vi "Build S1F1 Message Example.vi"(8 "error in":errorcluster) -> (0 "error out":errorcluster, 3 "SECS Packet":T1)   [LabVIEW 2016]
uses:
  Com/SECS Equipment/Data Def/Com_SECS Equipment _SECS Packet.ctl
  Com/SECS Equipment/Data Def/Com_SECS Equipment _Message Type.ctl
  Com/SECS Equipment/Data Def/Com_SECS Equipment _Protocol Type.ctl
  Com/SECS Equipment/Data Def/Com_SECS Equipment _Stream Type.ctl
  Com/SECS Equipment/Data Def/Com_SECS Equipment _Build Message Setting.ctl
  Com/SECS Equipment/Data Message/Com_SECS Equipment _Data Message_List.vi
  Com/SECS Equipment/Data Message/Com_SECS Equipment _Data Message_Boolean.vi
  Com/SECS Equipment/Data Message/Com_SECS Equipment _Data Message_F4.vi
  Com/SECS Equipment/Data Message/Com_SECS Equipment _Data Message_F8.vi
  Com/SECS Equipment/Data Message/Com_SECS Equipment _Data Message_Binary.vi
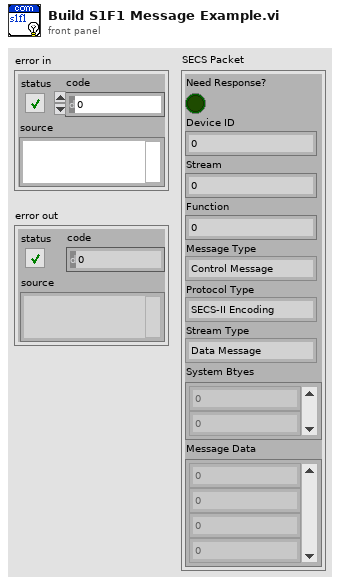
[diagram p1: front panel]
types:
  T1 = typedef "Com_SECS Equipment _SECS Packet.ctl" = cluster{"Need Response?":bool, "Device ID":u16, "Stream":u8, "Function":u8, "Message Type":T2, "Protocol Type":T3, "Stream Type":T4, "System Btyes":u8[], "Message Data":u8[]}
  T2 = typedef "Com_SECS Equipment _Message Type.ctl" = enum16{"Control Message", "Data Message"}
  T3 = typedef "Com_SECS Equipment _Protocol Type.ctl" = enum16{"SECS-II Encoding", "Reserved"}
  T4 = typedef "Com_SECS Equipment _Stream Type.ctl" = enum16{"Data Message", "Select.req", "Select.rsp", "Deselect.req", "Deselect.rsp", "Linktest.req", "Linktest.rsp", "Reject.req", "Separate.req", "Reserve"}
  T5 = typedef "Com_SECS Equipment _Build Message Setting.ctl" = cluster{"Stream":u8, "Function":u8, "Need Response?":bool}
  T6 = typedef "Com_SECS Equipment _Message Data.ctl" = cluster{"Index":i32, "Data Item Format":T7, "Format Code":T8, "Parent Index":i32, "Child Index":i32[], "Data":variant}
  T7 = typedef "Com_SECS Equipment _Data Item Format.ctl" = enum16{"Data Type", "Value"}
  T8 = typedef "Com_SECS Equipment _Format Code.ctl" = enum16{"L", "A", "B", "Boolean", "J", "I1", "I2", "I4", "I8", "U1", "U2", "U4", "U8", "F4", "F8", "Char"}
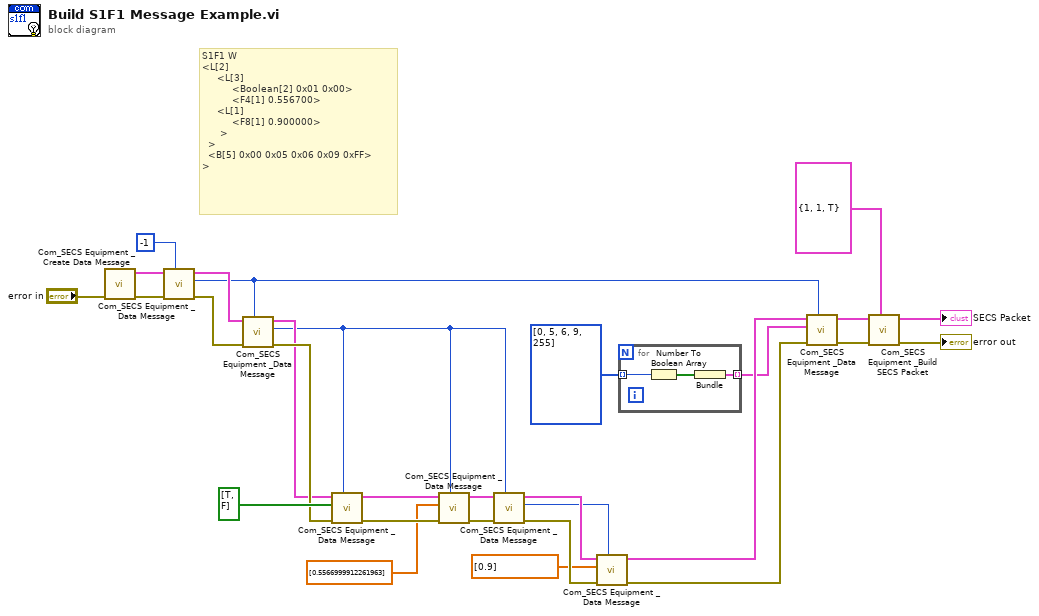
[diagram p0: block diagram]
diagram:
  # "S1F1 W\n<L[2]\n     <L[3]\n          <Boolean[2] 0x01 0x00>\n          <F4[1] 0.556700>\n     <L[1]\n          <F8[1] 0.900000>\n      >\n  >\n  <B[5] 0x00 0x05 0x06 0x09 0xFF>\n>"
  n1 = call "Com_SECS Equipment _Create Data Message.vi"("error in"="error in") -> ("error out"=w29:errorcluster, "Message Data"=w28:T6[])  [unwired: 9 in]
  n2 = call-poly "Com_SECS Equipment _Data Message.vi"("Parent Index"=-1, "error in"=w29, "Message Data In"=w28) -> ("error out"=w23:errorcluster, "Index"=w3:i32, "Message Data Out"=w22:T6[])  [unwired: 6 in]
  n3 = call-poly "Com_SECS Equipment _Data Message.vi"("Parent Index"=w3, "error in"=w23, "Message Data In"=w22) -> ("error out"=w21:errorcluster, "Index"=w2:i32, "Message Data Out"=w20:T6[])  [unwired: 6 in]
  n4 = call-poly "Com_SECS Equipment _Data Message.vi"("Parent Index"=w2, "error in"=w21, "Data"=bool[] [TRUE, FALSE], "Message Data In"=w20) -> ("error out"=w24:errorcluster, "Message Data Out"=w25:T6[])  [unwired: 6 in]
  n5 = call-poly "Com_SECS Equipment _Data Message.vi"("Parent Index"=w2, "error in"=w24, "Data"=sgl[] [0.5567], "Message Data In"=w25) -> ("error out"=w19:errorcluster, "Message Data Out"=w18:T6[])  [unwired: 6 in]
  n6 = call-poly "Com_SECS Equipment _Data Message.vi"("Parent Index"=w2, "error in"=w19, "Message Data In"=w18) -> ("error out"=w16:errorcluster, "Index"=w1:i32, "Message Data Out"=w15:T6[])  [unwired: 6 in]
  n7 = call-poly "Com_SECS Equipment _Data Message.vi"("Parent Index"=w1, "error in"=w16, "Data"=dbl[] [0.9], "Message Data In"=w15) -> ("error out"=w13:errorcluster, "Message Data Out"=w12:T6[])  [unwired: 6 in]
  n8 = for {
    tunnel: u8[] [0, 5, 6, 9, 255] -> [w32] mode=indexing
    tunnel: [w30] -> w10 mode=indexing
    n9 = Number To Boolean Array(number=w32) -> (Boolean array=w31:bool[])
    n10 = Bundle("Boolean array"=w31) -> (w30:cluster{"Boolean array":bool[]})  [unwired: 1 in]
  }
  n11 = call-poly "Com_SECS Equipment _Data Message.vi"("Parent Index"=w3, "error in"=w13, "Data Cluster"=w10, "Message Data In"=w12) -> ("error out"=w9:errorcluster, "Message Data Out"=w8:T6[])  [unwired: 6 in]
  n12 = call "Com_SECS Equipment _Build SECS Packet.vi"("Build Message Setting"=T5 {"Stream"=1, "Function"=1, "Need Response?"=TRUE}, "error in"=w9, "Message Data"=w8) -> ("error out"=→"error out":errorcluster, "SECS Packet"=→"SECS Packet":T1)  [unwired: 7 in]
